vi "GenerateHtmlDoc.vi"(8 "error in":errorcluster, 10 "Clear":bool, 11 "Vi":path) -> (0 "error out":errorcluster, 2 "VI Description":string, 3 "Html Path":path)   [LabVIEW 2020]
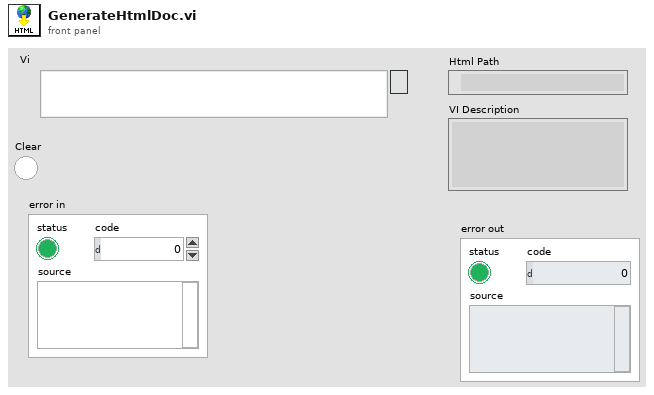
[diagram p1: front panel]
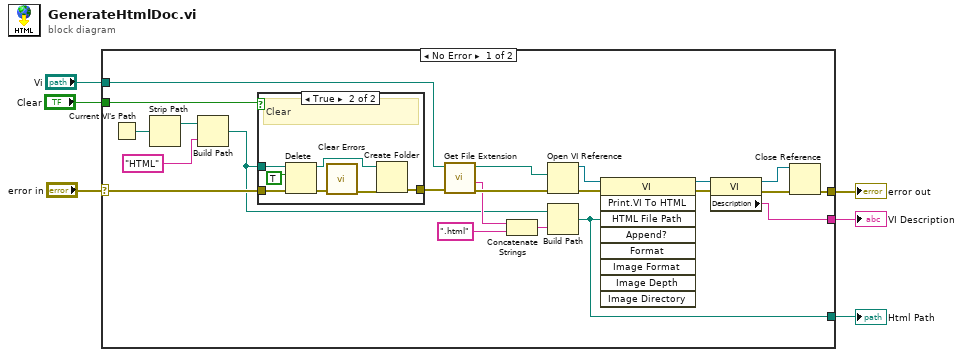
[diagram p0: block diagram]
diagram:
  n1 = case shown="No Error" "error in" {
    selector: "error in" -> [w14 w37]
    tunnel: "Vi" -> [w22 _]
    tunnel: [w16 w37] -> w5
    tunnel: [w15 _] -> w4
    tunnel: [w9 _] -> w2
    tunnel: "Clear" -> [w8 _]
    frame No Error {
      n2 = Current VI's Path() -> (path=w28:path)
      n3 = Strip Path(path=w28) -> (stripped path=w27:path)  [unwired: 1 out]
      n4 = Build Path(base path=w27, name or relative path="HTML") -> (appended path=w7:path)
      n5 = case shown="True" w8 {
        tunnel: w7 -> [_ w36]
        tunnel: [w29 w32] -> w23
        tunnel: w14 -> [w29 w31]
        frame False {
        }
        frame True {
          # "Clear"
          n6 = Delete(path (use dialog)=w36, entire hierarchy (F)=TRUE, error in=w31) -> (deleted path=w34:path, error out=w35:errorcluster)  [unwired: 2 in, 1 out]
          n7 = call <vilib>:"Clear Errors.vi"("error in (no error)"=w35) -> ("error out"=w33:errorcluster)  [unwired: 5 in, 1 out]
          n8 = Create Folder(path (use dialog)=w34, error in=w33) -> (error out=w32:errorcluster)  [unwired: 1 in, 2 out]
        }
      }
      n9 = call <vilib>:"Get File Extension.vi"("error in (no error)"=w23, "file"=w22) -> ("error out"=w20:errorcluster, "filename without extension"=w19:string, "dup file"=w21:path)  [unwired: 5 in, 2 out]
      n10 = Concatenate Strings(w19, ".html") -> (w18:string)
      n11 = Open VI Reference(vi path=w21, error in (no error)=w20) -> (vi reference=w24:refnum<vi>, error out=w25:errorcluster)  [unwired: 4 in]
      n12 = Build Path(base path=w7, name or relative path=w18) -> (appended path=w15:path)
      n13 = invoke class="VI" method="Print.VI To HTML"(reference=w24, error in=w25, "HTML File Path"=w15) -> (reference out=w13:refnum<vi>, error out=w12:errorcluster)  [unwired: 6 in, 7 out]
      n14 = property class="VI"(reference=w13, error in=w12) -> (reference out=w11:refnum<vi>, error out=w10:errorcluster, "Description"=w9:string)
      n15 = Close Reference(reference=w11, error in (no error)=w10) -> (error out=w16:errorcluster)
    }
    frame Error {
    }
  }
  "Html Path" <- w4
  "error out" <- w5
  "VI Description" <- w2
